vi "Ke2400 Enable.vi"(8 "error in (no error)":errorcluster, 10 "ON/OFF":bool, 11 "VISA In":refnum<visa-resource-name>) -> (0 "error out":errorcluster, 3 "VISA Out":refnum<visa-resource-name>)   [LabVIEW 2017]
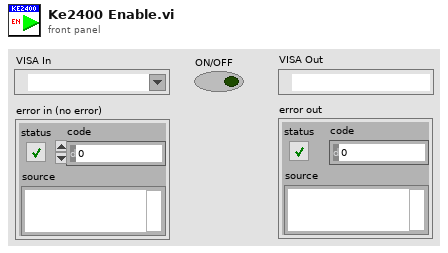
[diagram p1: front panel]
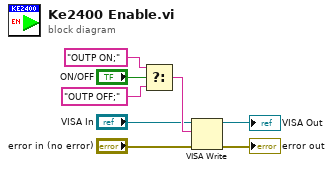
[diagram p0: block diagram]
diagram:
  n1 = Select(t="OUTP ON;", s="ON/OFF", f="OUTP OFF;") -> (s? t:f=w3:string)
  n2 = VISA Write(VISA resource name="VISA In", write buffer=w3, error in (no error)="error in (no error)") -> (VISA resource name out=→"VISA Out":refnum<visa-resource-name>, error out=→"error out":errorcluster)  [unwired: 1 out]
